vi "EncoderData_Receiver.vi"(4 "Option":i32, 5 "Timeout":i32=10000, 6 "SecondaryDataVIRef":refnum<vi>, 10 "EncoderData queue in":refnum<queue>, 11 "Gage CtrlQueue in":refnum<queue>) -> (0 "error out":errorcluster, 3 "PositionArray":dbl[][](array[numeric]))   [LabVIEW 2014]
uses:
  <instrlib>/GenericDAQ/VI/GenericDAQ_Ctrl_Queue.ctl
  <instrlib>/GenericDAQ/VI/GenericDAQ_State.ctl
  <vilib>/Utility/error.llb/Error Cluster From Error Code.vi
  <vilib>/ErrorRing/Error Ring.xnode
  <instrlib>/GenericDAQ/GenericDAQ.lvlib
panel:
  out "ctr":i32
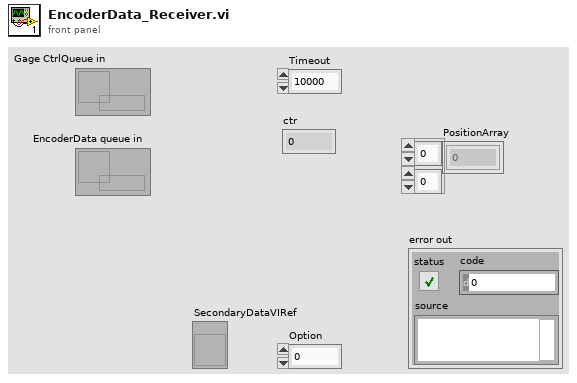
[diagram p1: front panel]
types:
  T1 = typedef "GenericDAQ.lvlib/GenericDAQ_Ctrl_Queue.ctl" = cluster{"GenericDAQ State":T2, "Variant":variant}
  T2 = typedef "GenericDAQ.lvlib/GenericDAQ_State.ctl" = enum16{"Enumerate", "Open", "Close", "CloseAll", "Reset", "Quit", "==Settings==", "SetAcquisition_", "SetChannels_", "SetTrigger_", "SetAnalogTrigDetector_", "SetSegment#_", "SetAll_AcquChTrig_", "fConfigurate", "fStart", "GetStatus", "_WaitForDone/Idle", "_GetData", "GetAcquisition", "GetChannels", "GetTrigger", "GetAll_AcquChTrig", "Abort", "==Messaging==", "_PushDataOut", "GetStat_", "GetConfig_", "==ModeSetup==", "SetSignalBuffer_", "SetMode_", "SetSecondaryDataRef._", "SetDynamicBuffer_", "==AnalogOut==", "GetChannelCount_AO", "fStart_AO", "SetChEnable_AO", "SetConfig_AO", "SetFuncData_AO", "SetOffset_AO_", "SetMasterNode_AO", "SetStates_AO", "SetSymetry_AO", "SetTriggerSource_AO", "==Trigger==", "ManualTrigger", "===Sync===", "LineStart", "LineEnd", "FrameStart", "FrameEnd", "EOL_PassThrough", "SOL_PassThrough"}
  T3 = cluster{"tickcount":u32, "Position":dbl[][], "Flag":enum16{"Normal", "MultiRecStart", "MultiRecEnd", "Reserved1", "Reserved2", "Reserved3"}}
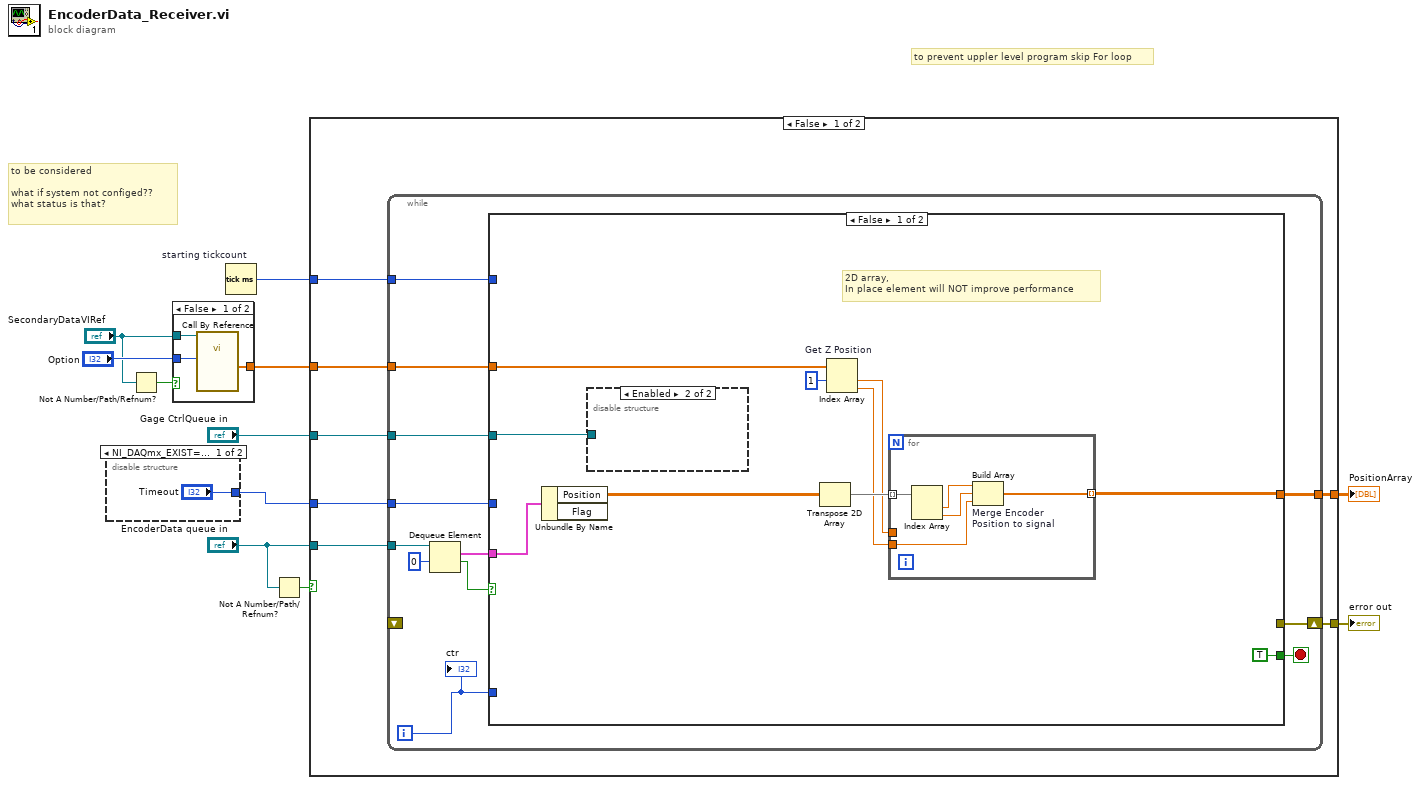
[diagram p0: block diagram]
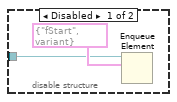
[diagram p3: hidden frame]
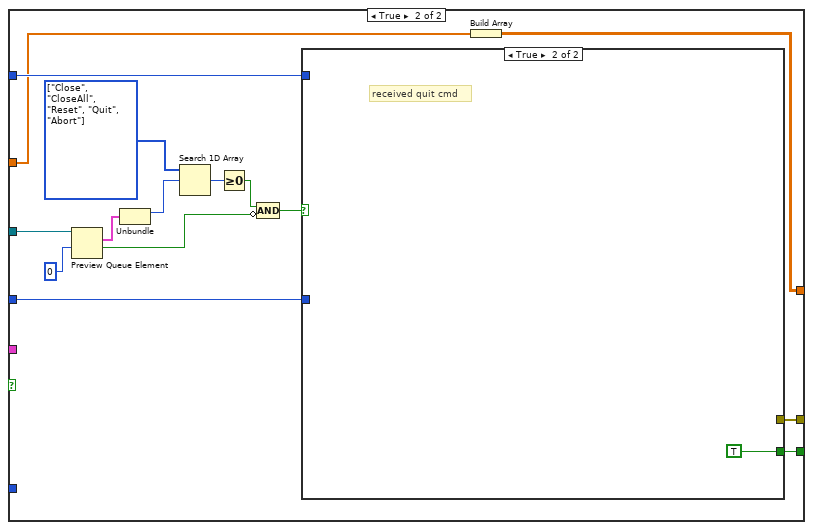
[diagram p4: hidden frame]
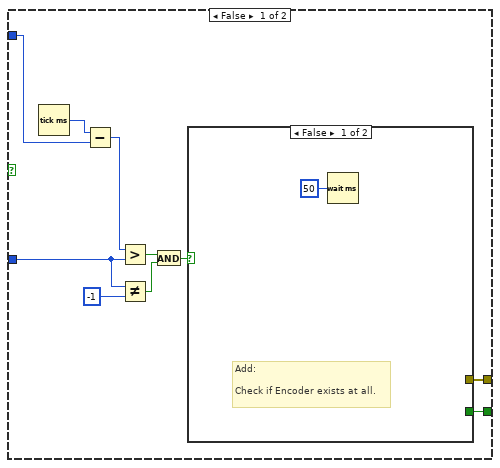
[diagram p5: hidden frame]
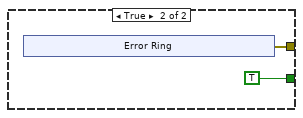
[diagram p6: hidden frame]
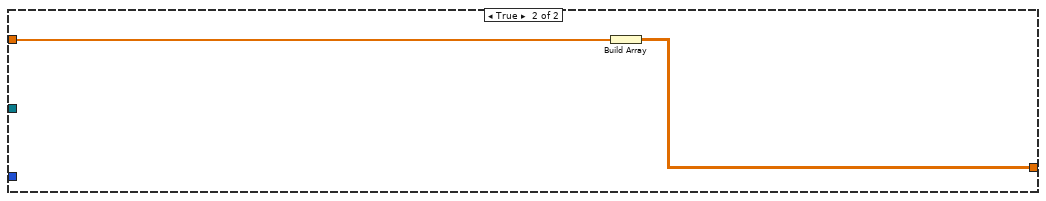
[diagram p7: hidden frame]
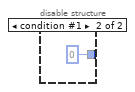
[diagram p8: hidden frame]
diagram:
  # "to prevent uppler level program skip For loop"
  # "to be considered \n\nwhat if system not configed??\nwhat status is that?"
  n1 = disable-structure shown="NI_DAQmx_EXIST==TRUE" {
    disable-tunnel: ["Timeout" 0 ("Timeout")] -> w7
    frame condition #0 (active) {
    }
    frame condition #1 {
    }
  }
  n2 = Not A Number/Path/Refnum?(number/path/refnum="SecondaryDataVIRef") -> (NaN/Path/Refnum?=w4:bool)
  n3 = case shown="False" w4 {
    tunnel: [w16 _] -> w1
    tunnel: "SecondaryDataVIRef" -> [w15 _]
    tunnel: "Option" -> [w14 _]
    frame False {
      n4 = call-by-ref "?"(reference=w15, "Option"=w14) -> ("SecondaryData"=w16:dbl[])  [unwired: 11 in, 2 out]
    }
    frame True {
    }
  }
  n5 = Tick Count (ms) "starting tickcount"() -> (millisecond timer value=w10:u32)
  n6 = Not A Number/Path/Refnum?(number/path/refnum="EncoderData queue in") -> (NaN/Path/Refnum?=w6:bool)
  n7 = case shown="False" w6 {
    tunnel: "EncoderData queue in" -> [w23 _]
    tunnel: "Gage CtrlQueue in" -> [w22 _]
    tunnel: w10 -> [w21 _]
    tunnel: [w20 _] -> w9
    tunnel: [w19 w88] -> w8
    tunnel: w7 -> [w18 _]
    tunnel: w1 -> [w17 w87]
    frame False {
      n8 = while {
        tunnel: w23 -> [w34]
        tunnel: [w31] -> w19
        tunnel: w22 -> [w30]
        tunnel: w21 -> [w29]
        shift-right: [w27] -> w20
        shift-left: _ -> [_]
        tunnel: w18 -> [w26]
        tunnel: w17 -> [w24]
        i -> [w25]
        stop <- w28 stop-if-true
        n9 = Dequeue Element(queue=w34, timeout in ms (-1)=0) -> (element=w33:T3, timed out?=w35:bool)  [unwired: 1 in, 2 out]
        n10 = case shown="False" w35 {
          tunnel: w33 -> [w44 _]
          tunnel: [w43 w54] -> w31
          tunnel: w30 -> [w36 w60]
          tunnel: w29 -> [_ w58]
          tunnel: [TRUE w57] -> w28
          tunnel: [_ w56] -> w27
          tunnel: w26 -> [_ w55]
          tunnel: w25 -> [_ _]
          tunnel: w24 -> [w39 w53]
          frame False {
            # "2D array,\nIn place element will NOT improve performance"
            n11 = Unbundle By Name(w44) -> ("Position"=w45:dbl[][])  [unwired: 1 out]
            n12 = disable-structure shown="Enabled" {
              disable-tunnel: w36 -> [w46 _]
              frame Disabled {
                n13 = Enqueue Element(queue=w46, element=T1 {"GenericDAQ State"=enum."fStart", "Variant"=variant}) -> ()  [unwired: 2 in, 3 out]
              }
              frame Enabled {
              }
            }
            n14 = Transpose 2D Array(2D array=w45) -> (transposed array=w42:dbl[][])
            n15 = Index Array "Get Z Position"(array=w39, index #1=1 ("index")) -> (element #1=w40:dbl, element #2=w37:dbl)  [unwired: 1 in]
            n16 = for {
              tunnel: w42 -> [w51] mode=indexing
              tunnel: [w50] -> w43 mode=indexing
              tunnel: w40 -> [_]
              tunnel: w37 -> [w49]
              n17 = Index Array(array=w51) -> (element #1=w52:dbl, element #2=w48:dbl)  [unwired: 2 in]
              n18 = Build Array "Merge Encoder \nPosition to signal"(w52, w48, w49) -> (w50:dbl[])
            }
          }
          frame True {
            w64 = T2[] [enum."Close", enum."CloseAll", enum."Reset", enum."Quit", enum."Abort"] items=["Enumerate", "Open", "Close", "CloseAll", "Reset", "Quit", "==Settings==", "SetAcquisition_", "SetChannels_", "SetTrigger_", "SetAnalogTrigDetector_", "SetSegment#_", "SetAll_AcquChTrig_", "fConfigurate", "fStart", "GetStatus", "_WaitForDone/Idle", "_GetData", "GetAcquisition", "GetChannels", "GetTrigger", "GetAll_AcquChTrig", "Abort", "==Messaging==", "_PushDataOut", "GetStat_", "GetConfig_", "==ModeSetup==", "SetSignalBuffer_", "SetMode_", "SetSecondaryDataRef._", "SetDynamicBuffer_", "==AnalogOut==", "GetChannelCount_AO", "fStart_AO", "SetChEnable_AO", "SetConfig_AO", "SetFuncData_AO", "SetOffset_AO_", "SetMasterNode_AO", "SetStates_AO", "SetSymetry_AO", "SetTriggerSource_AO", "==Trigger==", "ManualTrigger", "===Sync===", "LineStart", "LineEnd", "FrameStart", "FrameEnd", "EOL_PassThrough", "SOL_PassThrough"]
            n19 = Preview Queue Element(queue=w60, timeout in ms (-1)=0) -> (element=w62:T1, timed out?=w63:bool)  [unwired: 1 in, 2 out]
            n20 = Unbundle(w62) -> ("GenericDAQ State"=w67:T2)  [unwired: 1 out]
            n21 = Search 1D Array(1D array=w64, element=w67) -> (index of element=w65:i32)  [unwired: 1 in]
            n22 = Greater Or Equal To 0?(x=w65) -> (x >= 0?=w66:bool)
            n23 = Compound Arithmetic op=AND(w66, invert w63) -> (w59:bool)
            n24 = case shown="True" w59 {
              tunnel: w58 -> [w76 _]
              tunnel: [w74 TRUE] -> w57
              tunnel: [w73 _] -> w56
              tunnel: w55 -> [w68 _]
              frame False {
                n25 = Tick Count (ms)() -> (millisecond timer value=w77:u32)
                n26 = Subtract(x=w77, y=w76) -> (x-y=w75:u32)
                n27 = Greater?(x=w75, y=w68) -> (0:w72:bool)
                n28 = Not Equal?(x=w68, y=-1) -> (x != y?=w70:bool)
                n29 = And(x=w72, y=w70) -> (x .and. y?=w71:bool)
                n30 = case shown="False" w71 {
                  tunnel: [_ TRUE] -> w74
                  tunnel: [_ w79] -> w73
                  frame False {
                    # "Add:\n\nCheck if Encoder exists at all."
                    n31 = Wait (ms)(milliseconds to wait=u32 50) -> ()  [unwired: 1 out]
                  }
                  frame True {
                    n32 = xnode "Error Ring"() -> ("error out"=w79:errorcluster)
                  }
                }
              }
              frame True {
                # "received quit cmd"
              }
            }
            n33 = Build Array(w53) -> (w54:dbl[][])
          }
        }
        "ctr" <- w25
      }
    }
    frame True {
      n34 = Build Array(w87) -> (w88:dbl[][])
    }
  }
  "PositionArray" <- w8
  "error out" <- w9
